vi "Wii_Coords.vi"(11 "error in (no error)":errorcluster) -> (2 "Raw X Values":i32[](array[numeric]), 3 "Raw Y Values":i32[](array[numeric]), 4 "X Values":sgl[](array[numeric]), 6 "Y Values":sgl[](array[numeric]), 8 "Sizes":i32[](array[numeric]), 13 "B":bool, 14 "Home":bool, 15 "error out":errorcluster)   [LabVIEW 2011]
uses:
  libs/experiments 2/Action Engines/AE Access VIs/AE - Bluetooth ButtonAccData.vi
  libs/experiments 2/Action Engines/AE Access VIs/AE - Bluetooth IRData.vi
panel:
  # "Press \"Home\" for STOP"
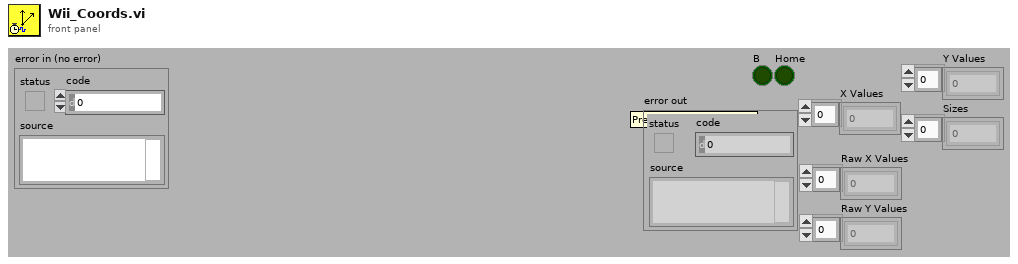
[diagram p1: front panel]
types:
  T1 = typedef "WiimoteState.ctl" = cluster{"X":sgl, "Y":sgl, "Z":sgl, "A":bool, "B":bool, "Down":bool, "Home":bool, "Left":bool, "Minus":bool, "One":bool, "Plus":bool, "Right":bool, "Two":bool, "Up":bool, "error out":errorcluster}
  T2 = typedef "WiimoteState(IR).ctl" = cluster{"Mode":u8, "IR State":bool[], "X Values":sgl[], "Y Values":sgl[], "Raw X Values":i32[], "Raw Y Values":i32[], "Sizes":i32[], "X Midpoint":sgl, "Y Midpoint":sgl}
  T3 = typedef "LVAllMonitorsDisplayTypeDef.ctl" = cluster{"Bounds":cluster{"Left":i16, "Top":i16, "Right":i16, "Bottom":i16}, "Depth":i16}[]
  T4 = cluster{"Bounds":cluster{"Left":i16, "Top":i16, "Right":i16, "Bottom":i16}, "Depth":i16}
  T5 = cluster{"Left":i16, "Top":i16, "Right":i16, "Bottom":i16}
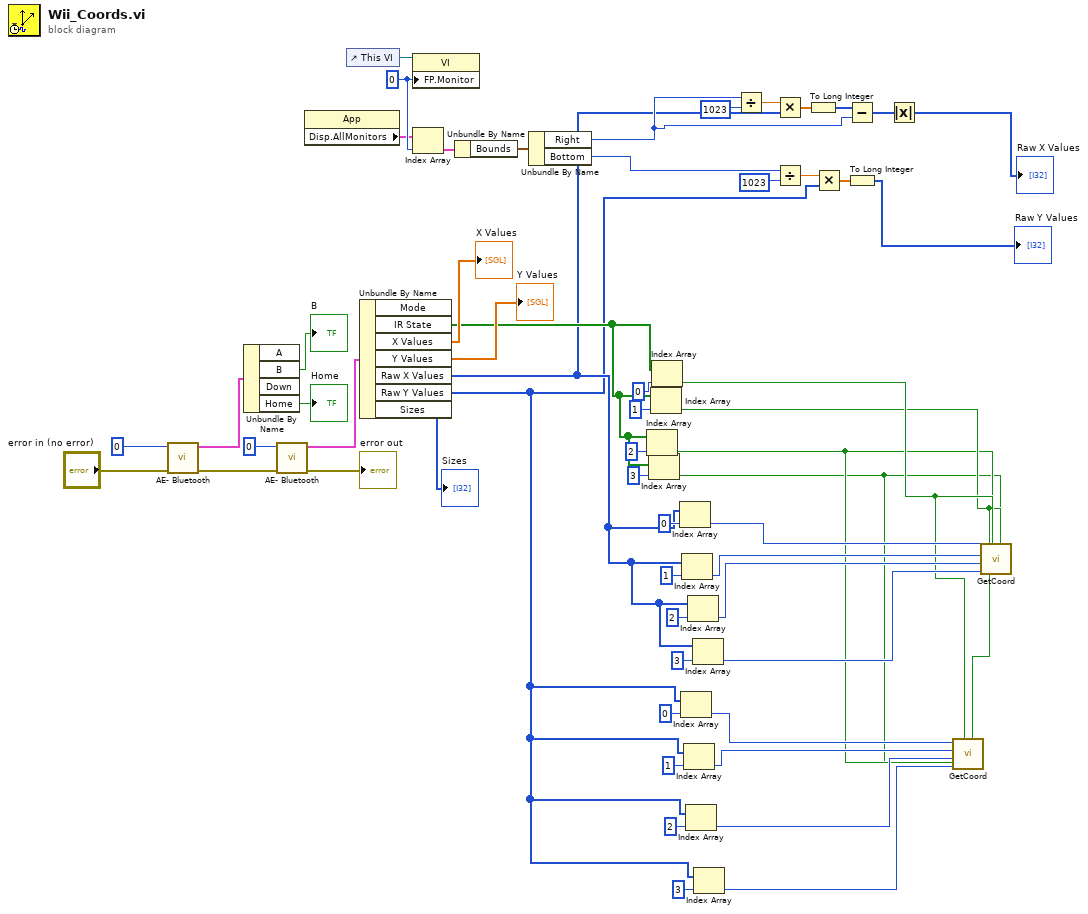
[diagram p0: block diagram]
diagram:
  w48 = u16 0 ("Front Panel Window:Monitor")
  n1 = call-poly "AE- Bluetooth.vi"("error in (no error)"="error in (no error)", "Wiimote"=0) -> ("error out"=w53:errorcluster, "Wiimote State"=w52:T1)  [unwired: 8 in]
  n2 = Unbundle By Name(w52) -> ("B"=→"B":bool, "Home"=→"Home":bool)  [unwired: 2 out]
  n3 = call-poly "AE- Bluetooth.vi"("error in (no error)"=w53, "Wiimote"=0) -> ("error out"=→"error out":errorcluster, "IRState"=w54:T2)  [unwired: 8 in]
  n4 = property class="App"() -> ("Disp.AllMonitors"=w47:T3)  [unwired: 2 in, 2 out]
  n5 = control-ref of="This VI"() -> (w50:refnum<vi>)
  n6 = Unbundle By Name(w54) -> ("IR State"=w21:bool[], "X Values"=→"X Values":sgl[], "Y Values"=→"Y Values":sgl[], "Raw X Values"=w4:i32[], "Raw Y Values"=w3:i32[], "Sizes"=→"Sizes":i32[])  [unwired: 1 out]
  n7 = property class="VI"(reference=w50, "FP.Monitor"=w48) -> ()  [unwired: 1 in, 2 out]
  n8 = Index Array(array=w47, index=w48) -> (element=w49:T4)
  n9 = Unbundle By Name(w49) -> ("Bounds"=w46:T5)
  n10 = Unbundle By Name(w46) -> ("Right"=w31:i16, "Bottom"=w32:i16)
  n11 = Index Array(array=w21, index=2) -> (element=w7:bool)
  n12 = Index Array(array=w21, index=3) -> (element=w6:bool)
  n13 = Index Array(array=w21, index=1) -> (element=w8:bool)
  n14 = Index Array(array=w21, index=0) -> (element=w9:bool)
  n15 = Index Array(array=w4, index=0) -> (element=w17:i32)
  n16 = Index Array(array=w3, index=0) -> (element=w13:i32)
  n17 = Index Array(array=w4, index=1) -> (element=w16:i32)
  n18 = Index Array(array=w3, index=1) -> (element=w12:i32)
  n19 = Index Array(array=w3, index=2) -> (element=w11:i32)
  n20 = Index Array(array=w4, index=2) -> (element=w15:i32)
  n21 = Index Array(array=w4, index=3) -> (element=w14:i32)
  n22 = Index Array(array=w3, index=3) -> (element=w10:i32)
  n23 = Divide(x=w31, y=i16 1023) -> (x/y=w39:dbl)
  n24 = Multiply(x=w39, y=w4) -> (x*y=w38:dbl[])
  n25 = Divide(x=w32, y=i16 1023) -> (x/y=w36:dbl)
  n26 = To Long Integer(number=w38) -> (32bit integer=w34:i32[])
  n27 = Multiply(x=w36, y=w3) -> (x*y=w35:dbl[])
  n28 = Subtract(x=w34, y=w31) -> (x-y=w33:i32[])
  n29 = To Long Integer(number=w35) -> (32bit integer=→"Raw Y Values":i32[])
  n30 = Absolute Value(x=w33) -> (abs(x)=→"Raw X Values":i32[])
  n31 = call "GetCoord.vi"(4:"4"=w6, 5:"2"=w8, 6:"3"=w7, 7:"1"=w9, 8:"4"=w10, 9:"3"=w11, 10:"2"=w12, 11:"1"=w13) -> ()  [unwired: 1 in, 3 out]
  n32 = call "GetCoord.vi"(4:"4"=w6, 5:"2"=w8, 6:"3"=w7, 7:"1"=w9, 8:"4"=w14, 9:"3"=w15, 10:"2"=w16, 11:"1"=w17) -> ()  [unwired: 1 in, 3 out]
